vi "Dynamic Terminals.vi"() -> ()   [LabVIEW 2023]
doc: "This example demonstrates dynamic terminals with LabVIEW classes.\n\nRefer to the LabVIEW Help for more information about LabVIEW object-oriented programming."
uses:
  Class Alpha/Class Alpha.lvclass
  Class Beta/Class Beta.lvclass
  Class Gamma/Class Gamma.lvclass
  Class Delta/Class Delta.lvclass
panel:
  out "Class Alpha out 5":refnum<class "Class Alpha.lvclass">
  out "Class Alpha out 4":refnum<class "Class Alpha.lvclass">
  out "Class Alpha out 3":refnum<class "Class Alpha.lvclass">
  in  "Class Delta.lvclass 2":refnum<class "Class Delta.lvclass">
  in  "Class Gamma.lvclass 2":refnum<class "Class Gamma.lvclass">
  in  "Class Beta.lvclass 2":refnum<class "Class Beta.lvclass">
  in  "Class Alpha.lvclass 2":refnum<class "Class Alpha.lvclass">
  out "Class Alpha out 2":refnum<class "Class Alpha.lvclass">
  in  "Class Delta.lvclass":refnum<class "Class Delta.lvclass">
  in  "Class Gamma.lvclass":refnum<class "Class Gamma.lvclass">
  in  "Class Beta.lvclass":refnum<class "Class Beta.lvclass">
  in  "Class Alpha.lvclass":refnum<class "Class Alpha.lvclass">
  out "Class Delta out":refnum<class "Class Delta.lvclass">
  out "Class Gamma out":refnum<class "Class Gamma.lvclass">
  out "Class Beta out":refnum<class "Class Beta.lvclass">
  out "Class Alpha out":refnum<class "Class Alpha.lvclass">
  # "Overview: This example contrasts dynamic and static terminals with LabVIEW classes.\nInstructions:\n1. Select View>>LabVIEW Class Hierarchy to see the inheritance chain of the four classes in this example.\n2. You do not need to run this VI.\n3. Open the block diagram and refer to the comments there."
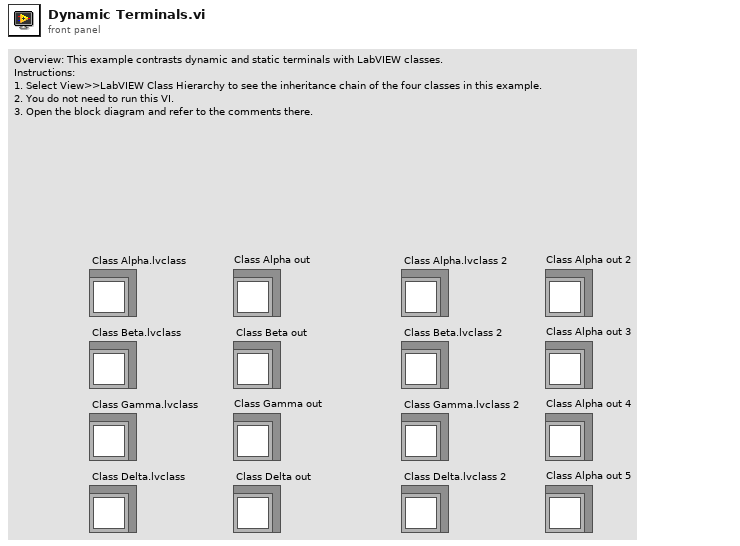
[diagram p1: front panel]
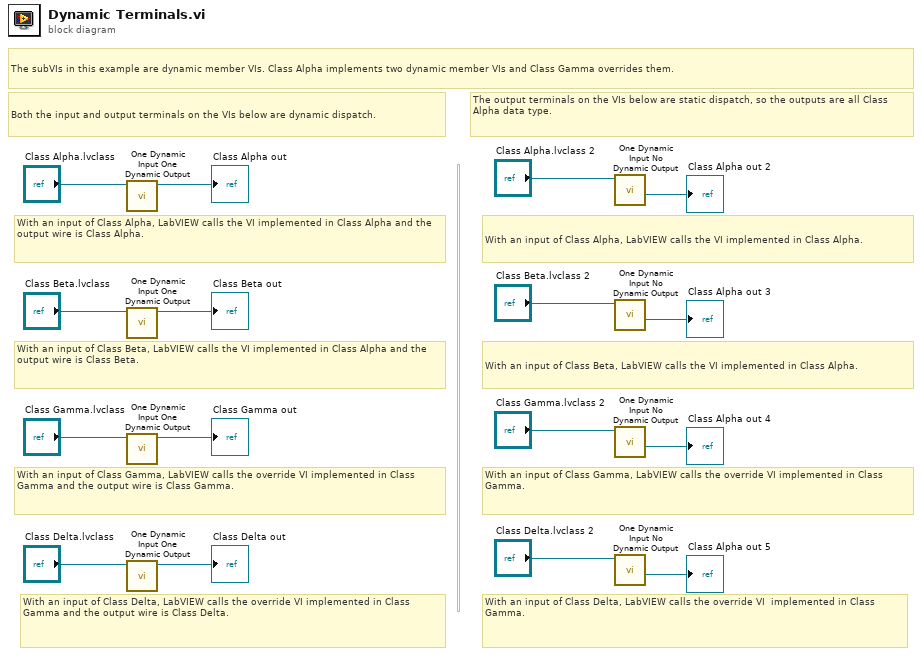
[diagram p0: block diagram]
diagram:
  # "The output terminals on the VIs below are static dispatch, so the outputs are all Class Alpha data type."
  # "With an input of Class Delta, LabVIEW calls the override VI  implemented in Class Gamma."
  # "With an input of Class Gamma, LabVIEW calls the override VI implemented in Class Gamma."
  # "With an input of Class Beta, LabVIEW calls the VI implemented in Class Alpha."
  # "With an input of Class Alpha, LabVIEW calls the VI implemented in Class Alpha."
  # "Both the input and output terminals on the VIs below are dynamic dispatch."
  # "With an input of Class Delta, LabVIEW calls the override VI implemented in Class Gamma and the output wire is Class Delta."
  # "With an input of Class Gamma, LabVIEW calls the override VI implemented in Class Gamma and the output wire is Class Gamma."
  # "With an input of Class Beta, LabVIEW calls the VI implemented in Class Alpha and the output wire is Class Beta."
  # "With an input of Class Alpha, LabVIEW calls the VI implemented in Class Alpha and the output wire is Class Alpha."
  # "The subVIs in this example are dynamic member VIs. Class Alpha implements two dynamic member VIs and Class Gamma overrides them."
  n1 = call-dynamic "One Dynamic Input One Dynamic Output.vi"("Class Alpha in"="Class Alpha.lvclass") -> ("Class Alpha out"=→"Class Alpha out":refnum<class "Class Alpha.lvclass">)  [unwired: 1 in, 9 out]
  n2 = call-dynamic "One Dynamic Input One Dynamic Output.vi"("Class Alpha in"="Class Beta.lvclass") -> ("Class Alpha out"=→"Class Beta out":refnum<class "Class Beta.lvclass">)  [unwired: 1 in, 9 out]
  n3 = call-dynamic "One Dynamic Input One Dynamic Output.vi"("Class Gamma in"="Class Gamma.lvclass") -> ("Class Gamma out"=→"Class Gamma out":refnum<class "Class Gamma.lvclass">)  [unwired: 1 in, 9 out]
  n4 = call-dynamic "One Dynamic Input One Dynamic Output.vi"("Class Gamma in"="Class Delta.lvclass") -> ("Class Gamma out"=→"Class Delta out":refnum<class "Class Delta.lvclass">)  [unwired: 1 in, 9 out]
  n5 = call-dynamic "One Dynamic Input No Dynamic Output.vi"("Class Alpha in"="Class Alpha.lvclass 2") -> ("Class Alpha out"=→"Class Alpha out 2":refnum<class "Class Alpha.lvclass">)  [unwired: 1 in, 9 out]
  n6 = call-dynamic "One Dynamic Input No Dynamic Output.vi"("Class Alpha in"="Class Beta.lvclass 2") -> ("Class Alpha out"=→"Class Alpha out 3":refnum<class "Class Alpha.lvclass">)  [unwired: 1 in, 9 out]
  n7 = call-dynamic "One Dynamic Input No Dynamic Output.vi"("Class Gamma in"="Class Gamma.lvclass 2") -> ("Class Alpha out"=→"Class Alpha out 4":refnum<class "Class Alpha.lvclass">)  [unwired: 1 in, 9 out]
  n8 = call-dynamic "One Dynamic Input No Dynamic Output.vi"("Class Gamma in"="Class Delta.lvclass 2") -> ("Class Alpha out"=→"Class Alpha out 5":refnum<class "Class Alpha.lvclass">)  [unwired: 1 in, 9 out]
